vi "SetDigitalPWMCommand.vi"(10 "Value":u8, 11 "Pin":u8) -> ()   [LabVIEW 2021]
uses:
  CommandType.ctl
panel:
  out "Command":T1
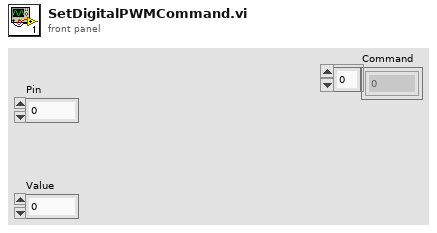
[diagram p1: front panel]
types:
  T1 = typedef "CommandType.ctl" = u8[]
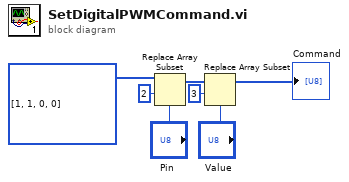
[diagram p0: block diagram]
diagram:
  n1 = Replace Array Subset(array=u8[] [1, 1, 0, 0], new element="Pin", index=2 ("indice")) -> (w4:u8[])
  n2 = Replace Array Subset(array=w4, new element="Value", index=3 ("indice")) -> (→"Command":u8[])
